vi "Add Transfers Buffers with Children.vi"(6 "Decimation":u64, 7 "buffer descriptor":T6={"buffer type"=enum."Engine", "plugin id"=-1, "group id"=-1, "transfer id"=-1, "offset"=0, "length"=-1}, 8 "error in (no error)":errorcluster, 9 "Transfer configuration":T1 {"channels"."string offset" format="%d bytes"}, 10 "parent tag":string, 11 "Application Data In":T8) -> (0 "error out":errorcluster, 3 "Application Data out":T8)   [LabVIEW 2017, in "DSF Core.lvlib"]
uses:
  DSF Core.lvlib
  Main VI/Application Data.ctl
  <vilib>/NI/Memory Manager/Classes/Pointer/Pointer.lvclass
  Buffer Reader/Queue Data.ctl
  Buffer Reader/Buffer Data.ctl
  Typedefs/DSF Data Type.ctl
  Typedefs/DSF Engine Channel Configuration.ctl
  Typedefs/DSF Settings Info.ctl
  Typedefs/DSF Byte Order.ctl
  Classes/Thread/Data Server/DSF Buffer Subset Descriptor.ctl
  Typedefs/DSF Buffer Type.ctl
  Typedefs/DSF Engine Framework Configuration.ctl
  Typedefs/DSF Engine Plugin Configuration.ctl
  Typedefs/DSF Timing Info.ctl
  Typedefs/DSF Engine Plugin Thread Configuration.ctl
  Typedefs/DSF Engine Transfer Group Configuration.ctl
  Typedefs/DSF Direction.ctl
  Typedefs/DSF Engine Transfer Configuration.ctl
  Typedefs/DSF Timeout Behavior.ctl
  ID to Tree Items/Tree Item Type.ctl
  Classes/Configuration/Required Buffer Size (Transfer).vi
  Classes/Configuration/Configuration Session.lvclass
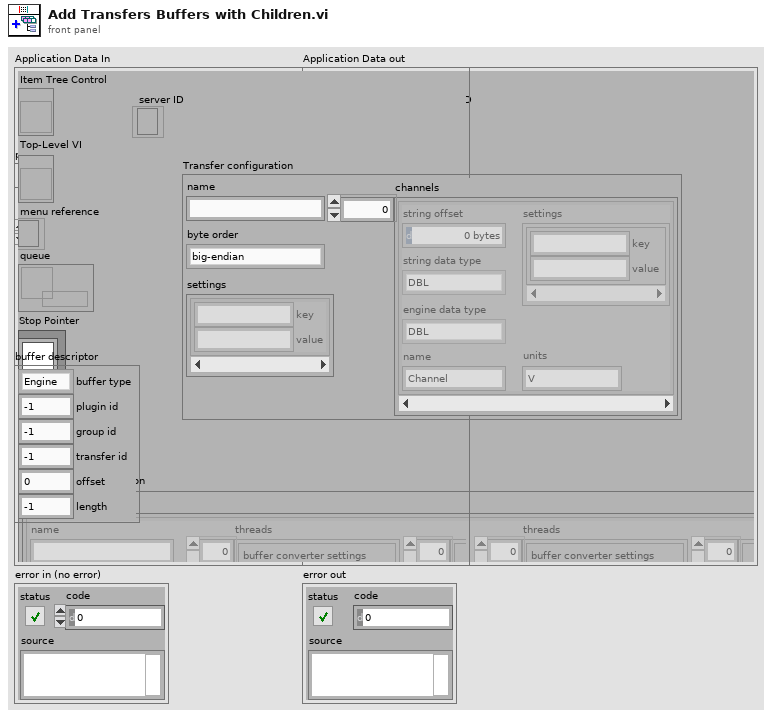
[diagram p1: front panel]
types:
  T1 = typedef "DSF Core.lvlib/DSF Engine Transfer Configuration.ctl" = cluster{"name":string, "byte order":T2, "settings":T3, "channels":T4[]}
  T2 = typedef "DSF Core.lvlib/DSF Byte Order.ctl" = enum8{"big-endian", "little-endian"}
  T3 = typedef "DSF Core.lvlib/DSF Settings Info.ctl" = cluster{"key":string, "value":string}[]
  T4 = typedef "DSF Core.lvlib/DSF Engine Channel Configuration.ctl" = cluster{"string offset":u64, "string data type":T5, "engine data type":T5, "name":string, "settings":T3, "units":string}
  T5 = typedef "DSF Core.lvlib/DSF Data Type.ctl" = enum8{"Bool", "SGL", "DBL", "I8", "I16", "I32", "I64", "U8", "U16", "U32", "U64"}
  T6 = typedef "DSF Core.lvlib/DSF Buffer Subset Descriptor.ctl" = cluster{"buffer type":T7, "plugin id":i32, "group id":i32, "transfer id":i32, "offset":u64, "length":i64}
  T7 = typedef "DSF Core.lvlib/DSF Buffer Type.ctl" = enum16{"Engine", "String"}
  T8 = typedef "DSF Core.lvlib/Application Data.ctl" = cluster{"Item Tree Control":refnum<vi>, "Top-Level VI":refnum<vi>, "menu reference":refnum<k9>, "queue":refnum<queue>, "Stop Pointer":refnum<class "Pointer.lvclass">, "Buffer Variant":variant, "Framework Configuration":T9, "server ID":refnum<k5>}
  T9 = typedef "DSF Core.lvlib/DSF Engine Framework Configuration.ctl" = cluster{"Plugins":T10[]}
  T10 = typedef "DSF Core.lvlib/DSF Engine Plugin Configuration.ctl" = cluster{"name":string, "components":string[], "cycle timing":T11, "threads":T12[], "Transfer Groups":T13[], "settings":T3}
  T11 = typedef "DSF Core.lvlib/DSF Timing Info.ctl" = cluster{"priority":u64, "decimation":u64, "offset":u64}
  T12 = typedef "DSF Core.lvlib/DSF Engine Plugin Thread Configuration.ctl" = cluster{"buffer converter settings":T3, "transceiver settings":T3, "custom settings":T3, "processor":i32, "priority offset":i16}
  T13 = typedef "DSF Core.lvlib/DSF Engine Transfer Group Configuration.ctl" = cluster{"name":string, "direction":T14, "cycle timing":T11, "thread index":i32, "settings":T3, "Transfers":T1[], "timeout behavior":T15}
  T14 = typedef "DSF Core.lvlib/DSF Direction.ctl" = enum8{"Tx", "Rx"}
  T15 = typedef "DSF Core.lvlib/DSF Timeout Behavior.ctl" = enum8{"Increment Late Count", "Throw Error"}
  T16 = typedef "DSF Core.lvlib/Buffer Data.ctl" = cluster{"decimation":u64, "avg bandwidth":dbl, "data type":T5, "units":string, "channels":T4[], "channel":bool, "engine (T) / string (F)":bool, "byte order":T2, "buffer descriptor":T6}
  T17 = typedef "DSF Core.lvlib/Tree Item Type.ctl" = enum16{"Framework", "Plugin Group", "Plugin", "Group", "Transfer", "Buffer", "Channel"}
  T18 = typedef "DSF Core.lvlib/Tree Item.ctl" = cluster{"Left Cell String":string, "Child Text":string[], "Child Tag":string, "Glyph Index":i32}
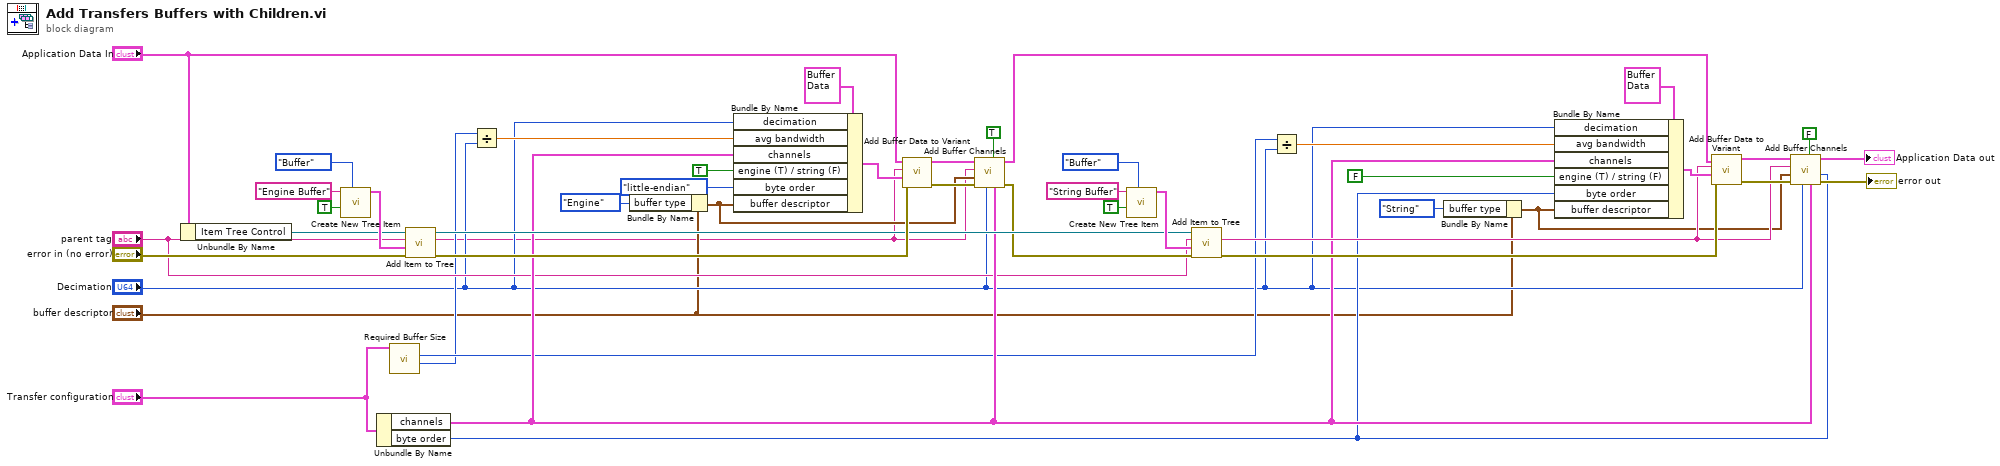
[diagram p0: block diagram]
diagram:
  n1 = Unbundle By Name("Application Data In") -> ("Item Tree Control"=w30:refnum<vi>)
  n2 = call "Create New Tree Item.vi"("Item Type"=Tree_Item_Type."Buffer", "found?"=TRUE, "Left Cell String"="Engine Buffer") -> ("Item"=w32:T18)  [unwired: 7 in, 1 out]
  n3 = Unbundle By Name("Transfer configuration") -> ("channels"=w16:T4[], "byte order"=w8:T2)
  n4 = call-poly "Required Buffer Size.vi"("Transfer Configuration in"="Transfer configuration") -> ("engine buffer size"=w9:u64, "string buffer size"=w14:u64)  [unwired: 7 in, 2 out]
  n5 = call "Add Item to Tree.vi"("error in (no error)"="error in (no error)", "Item"=w32, "parent tag"="parent tag", "TreeControl in"=w30) -> ("error out"=w44:errorcluster, "new item tag"=w2:string, "TreeControl out"=w39:refnum<vi>)  [unwired: 5 in]
  n6 = Divide(x=w9, y="Decimation") -> (x/y=w12:dbl)
  n7 = Bundle By Name(cluster="buffer descriptor", "buffer type"=DSF_Buffer_Type."Engine") -> (w3:T6)
  n8 = Bundle By Name(cluster=T16 {"decimation"=0, "avg bandwidth"=0.0, "data type"=enum."Bool", "units"="", "channels"=[], "channel"=FALSE, "engine (T) / string (F)"=FALSE, "byte order"=enum."big-endian", "buffer descriptor"={"buffer type"=enum."Engine", "plugin id"=0, "group id"=0, "transfer id"=0, "offset"=0, "length"=0}} ("Buffer data"), "decimation"="Decimation", "avg bandwidth"=w12, "channels"=w16, "engine (T) / string (F)"=TRUE, "byte order"=DSF_Byte_Order."little-endian", "buffer descriptor"=w3) -> (w43:T16)
  n9 = call "Add Buffer Data to Variant.vi"("error in (no error)"=w44, "Buffer data"=w43, "tag"=w2, "Application Data In in"="Application Data In") -> ("error out"=w28:errorcluster, "Application Data In out"=w29:T8)  [unwired: 6 in]
  n10 = call "Add Buffer Channels.vi"("channels"=w16, "engine (T) / string (F)"=TRUE, "Decimation"="Decimation", "error in (no error)"=w28, "buffer descriptor"=w3, "parent tag"=w2, "Application Data In"=w29) -> ("error out"=w27:errorcluster, "Application Data out"=w11:T8)  [unwired: 3 in]
  n11 = call "Create New Tree Item.vi"("Item Type"=Tree_Item_Type."Buffer", "found?"=TRUE, "Left Cell String"="String Buffer") -> ("Item"=w40:T18)  [unwired: 7 in, 1 out]
  n12 = call "Add Item to Tree.vi"("error in (no error)"=w27, "Item"=w40, "parent tag"="parent tag", "TreeControl in"=w39) -> ("error out"=w47:errorcluster, "new item tag"=w21:string)  [unwired: 5 in, 1 out]
  n13 = Divide(x=w14, y="Decimation") -> (x/y=w13:dbl)
  n14 = Bundle By Name(cluster="buffer descriptor", "buffer type"=DSF_Buffer_Type."String") -> (w1:T6)
  n15 = Bundle By Name(cluster=T16 {"decimation"=0, "avg bandwidth"=0.0, "data type"=enum."Bool", "units"="", "channels"=[], "channel"=FALSE, "engine (T) / string (F)"=FALSE, "byte order"=enum."big-endian", "buffer descriptor"={"buffer type"=enum."Engine", "plugin id"=0, "group id"=0, "transfer id"=0, "offset"=0, "length"=0}} ("Buffer data"), "decimation"="Decimation", "avg bandwidth"=w13, "channels"=w16, "engine (T) / string (F)"=FALSE, "byte order"=w8, "buffer descriptor"=w1) -> (w46:T16)
  n16 = call "Add Buffer Data to Variant.vi"("error in (no error)"=w47, "Buffer data"=w46, "tag"=w21, "Application Data In in"=w11) -> ("error out"=w23:errorcluster, "Application Data In out"=w25:T8)  [unwired: 6 in]
  n17 = call "Add Buffer Channels.vi"("byte order"=w8, "channels"=w16, "engine (T) / string (F)"=FALSE, "Decimation"="Decimation", "error in (no error)"=w23, "buffer descriptor"=w1, "parent tag"=w21, "Application Data In"=w25) -> ("error out"=→"error out":errorcluster, "Application Data out"=→"Application Data out":T8)  [unwired: 2 in]
